vi "SetDelay.vi"(8 "Mixer freq [MHz]":dbl, 9 "Output delay delta":dbl, 10 "Output delay":dbl, 11 "scope in":T1) -> (3 "scope out":T1)   [LabVIEW 2013]
uses:
  controls/scope_params_5782.ctl
  Utilities/Ticker/Ticker.lvclass
  Communication/Driver/RemoteConnection/RemoteConnection.lvclass
  Scope/controls/ScopeMode.ctl
  Config/FPGAref_5782.ctl
  FPGA/DataMode.ctl
  controls/5782_trigger_type.ctl
  FPGA/fpga_settings.ctl
  <vilib>/rvi/interface/common/niFpgaWaitOnOcc.vi
  <vilib>/Utility/error.llb/Error Cluster From Error Code.vi
  <vilib>/rvi/errors/niLvFpgaAdjustHostInterfaceError.vi
  <vilib>/rvi/FXPMathLib/FxpInterpret/XNode/nifxpmath_Interpret.xnode
  <vilib>/rvi/interface/nirviReadWriteControl/nirviReadWriteControl.xnode
  NiFpgaLv.dll
  <vilib>/rvi/interface/Simulation/niFpgaSimulationCallBeginRW.vi
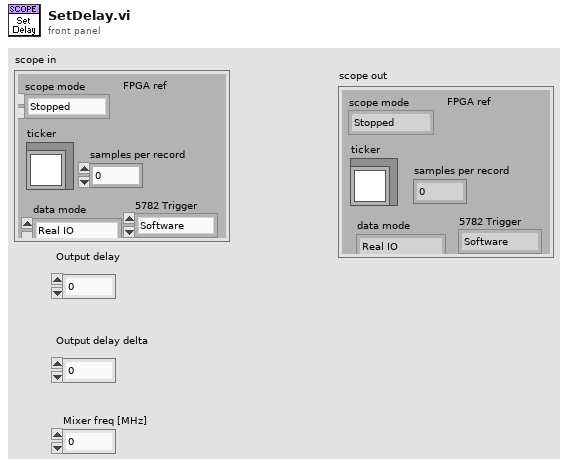
[diagram p1: front panel]
types:
  T1 = typedef "scope_params_5782.ctl" = cluster{"scope mode":T2, "ticker":refnum<class "Ticker.lvclass">, "samples per record":i32, "FPGA ref":T3, "data mode":T4, "5782 Trigger":T5, "Chart length":i32, "RemoteConnection":refnum<class "RemoteConnection.lvclass">, "last phase":dbl[]}
  T2 = typedef "ScopeMode.ctl" = enum16{"Stopped", "Single", "Running", "Continuous"}
  T3 = typedef "FPGAref_5782.ctl" = refnum<k20>
  T4 = typedef "DataMode.ctl" = enum16{"Real IO", "Simulated"}
  T5 = typedef "5782_trigger_type.ctl" = enum16{"Software", "Trigger input"}
  T6 = typedef "fpga_settings.ctl" = enum16{"Feedback Enable", "New FIR coeffs", "FIR shift", "Enable filter", "Set Downsample", "Downsample", "CIC Gain", "Record length", "Trigger samples", "Quiet time", "a_am", "b_am", "Use fixed delay", "fixed sin_fi", "fixed cos_fi", "Ki*Tau", "Kp", "Kd_Tau", "Fi_start", "Fi_delta", "DC_offs 0", "DC_offs 1", "DC_offs 2", "DC_offs 3", "Ki*Tau am", "Kp am", "Kd_Tau am", "Feedback AM"}
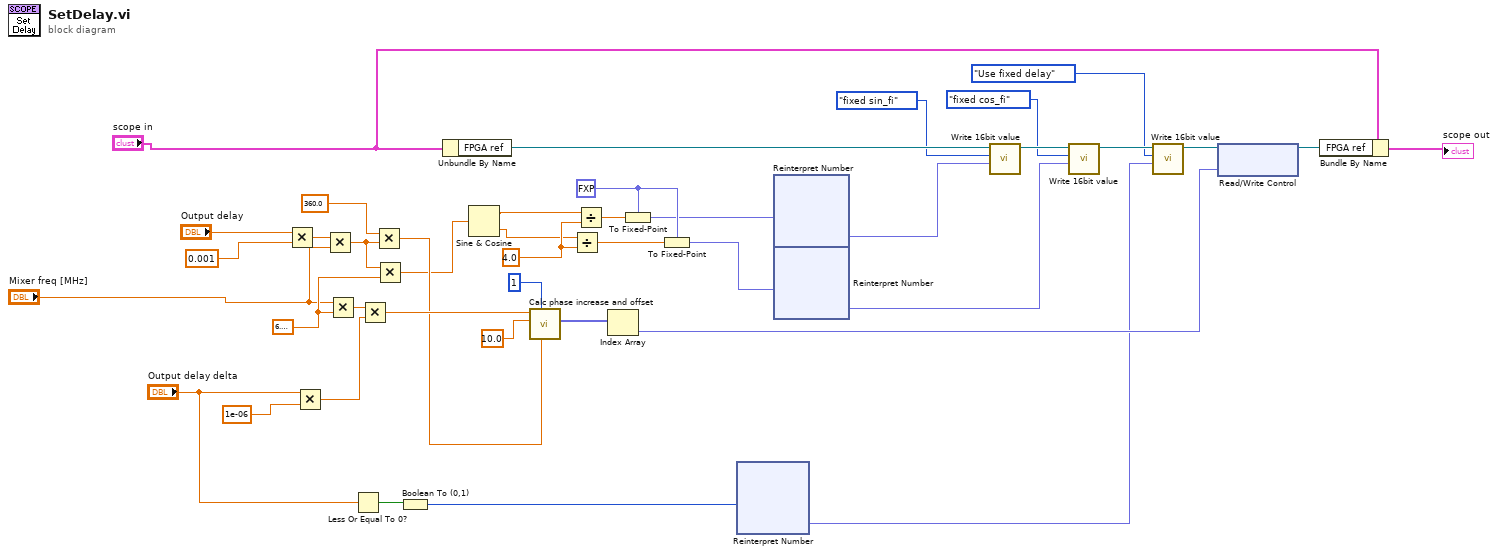
[diagram p0: block diagram]
diagram:
  w22 = 4.0 ("y")
  w23 = fxp<+/-,16,0> 0.0 ("fixed sin fi")
  w26 = 6.283185307179586
  n1 = Multiply(x="Output delay", y=0.001) -> (x*y=w32:dbl)
  n2 = Multiply(x="Output delay delta", y=1e-06) -> (x*y=w33:dbl)
  n3 = Multiply(x=w32, y="Mixer freq [MHz]") -> (x*y=w27:dbl)
  n4 = Multiply(x="Mixer freq [MHz]", y=w26) -> (x*y=w38:dbl)
  n5 = Less Or Equal To 0?(x="Output delay delta") -> (x <= 0?=w11:bool)
  n6 = Multiply(x=w38, y=w33) -> (x*y=w37:dbl)
  n7 = Multiply(x=360.0, y=w27) -> (x*y=w30:dbl)
  n8 = Multiply(x=w27, y=w26) -> (x*y=w25:dbl)
  n9 = Boolean To (0,1)(Boolean=w11) -> (0, 1=w10:i16)
  n10 = Unbundle By Name("scope in") -> ("FPGA ref"=w9:T3)
  n11 = Sine & Cosine(0:w25) -> (1:w21:dbl, 2:w18:dbl)
  n12 = call "Calc phase increase and offset.vi"("Phase offset (deg)"=w30, "# of DDS"=1, "fclk (MHz)"=10.0, "f_generated (MHz)"=w37) -> ("Phase out"=w29:fxp<+,64,64>[])  [unwired: 5 in, 2 out]
  n13 = Divide(x=w18, y=w22) -> (x/y=w19:dbl)
  n14 = Divide(x=w21, y=w22) -> (x/y=w20:dbl)
  n15 = Index Array(array=w29) -> (element=w24:fxp<+,64,64>)  [unwired: 1 in]
  n16 = To Fixed-Point(fixed-point type=w23, number=w20) -> (fixed-point=w13:fxp<+/-,16,0>)
  n17 = To Fixed-Point(fixed-point type=w23, number=w19) -> (fixed-point=w12:fxp<+/-,16,0>)
  n18 = xnode "Reinterpret Number"("x"=w10) -> ("y"=w4:fxp<+,16,16>)
  n19 = xnode "Reinterpret Number"("x"=w13) -> ("y"=w14:fxp<+,16,16>)
  n20 = xnode "Reinterpret Number"("x"=w12) -> ("y"=w5:fxp<+,16,16>)
  n21 = call "Write 16bit value.vi"("value"=w14, "FPGA Setting"=fpga_settings."fixed sin_fi", "FPGA ref"=w9) -> ("FPGA ref out"=w8:T3)  [unwired: 7 in, 1 out]
  n22 = call "Write 16bit value.vi"("value"=w5, "FPGA Setting"=fpga_settings."fixed cos_fi", "FPGA ref"=w8) -> ("FPGA ref out"=w7:T3)  [unwired: 7 in, 1 out]
  n23 = call "Write 16bit value.vi"("value"=w4, "FPGA Setting"=fpga_settings."Use fixed delay", "FPGA ref"=w7) -> ("FPGA ref out"=w6:T3)  [unwired: 7 in, 1 out]
  n24 = xnode "Read/Write Control"("FPGA VI Reference In"=w6, "delay phase"=w24) -> ("FPGA VI Reference Out"=w41:T3)  [unwired: 1 in, 1 out]
  n25 = Bundle By Name(cluster="scope in", "FPGA ref"=w41) -> (→"scope out":T1)
